vi "Draw Range Border.vi"(4 "Marker Options":T2={"Color"=16723218, "pen"={"Width"=2, "Style"=enum."Solid"}, "font"={"Font Name"="Arial", "Size"=16, "Strikeout?"=FALSE, "Italic?"=FALSE, "Underline?"=FALSE, "Outline?"=FALSE, "Shadow?"=FALSE, "Bold?"=FALSE, "FontColor"=0}, "caption"=""}, 6 "Type":T1, 7 "picture":picture, 9 "end Coords":T3, 10 "Plot Bounds":T4, 11 "Start Coords":T3) -> (5 "new picture":picture)   [LabVIEW 2014, in "Graph Extensions.lvlib"]
uses:
  Graph Extensions.lvlib
  <vilib>/Utility/miscctls.llb/LVRectTypeDef.ctl
  <vilib>/Utility/miscctls.llb/LVPoint32TypeDef.ctl
  controls/MarkerOptions.ctl
  controls/markerType.ctl
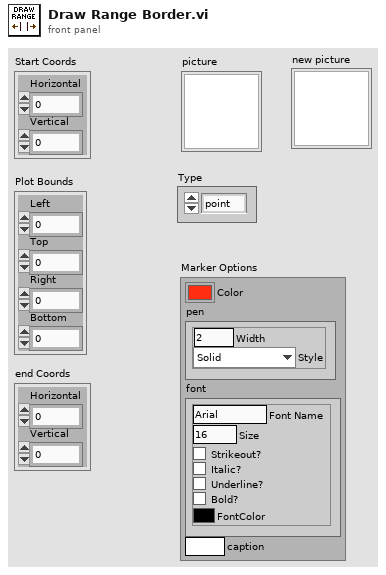
[diagram p1: front panel]
types:
  T1 = typedef "Graph Extensions.lvlib/markerType.ctl" = enum16{"point", "arrow", "horiz", "vert", "vert range", "horiz range", "box"}
  T2 = typedef "Graph Extensions.lvlib/MarkerOptions.ctl" = cluster{"Color":u32, "pen":cluster{"Width":u16, "Style":enum32{"Solid", "Dash", "Dot", "DashDot", "DashDotDot"}}, "font":cluster{"Font Name":string, "Size":i16, "Strikeout?":bool, "Italic?":bool, "Underline?":bool, "Outline?":bool, "Shadow?":bool, "Bold?":bool, "FontColor":u32}, "caption":string}
  T3 = typedef "LVPoint32TypeDef.ctl" = cluster{"Horizontal":i32, "Vertical":i32}
  T4 = typedef "LVRectTypeDef.ctl" = cluster{"Left":i16, "Top":i16, "Right":i16, "Bottom":i16}
  T5 = cluster{"Width":u16, "Style":enum32{"Solid", "Dash", "Dot", "DashDot", "DashDotDot"}}
  T6 = cluster{"left":i16, "top":i16, "right":i16, "bottom":i16}
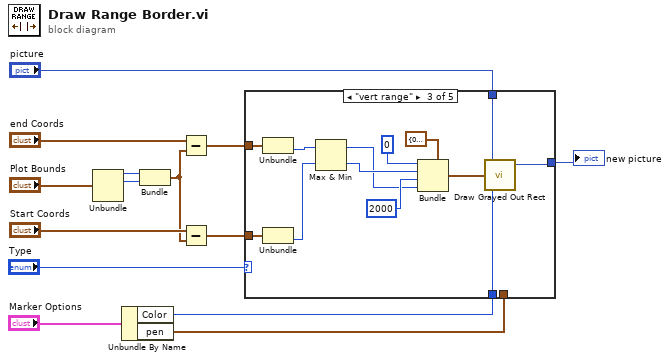
[diagram p0: block diagram]
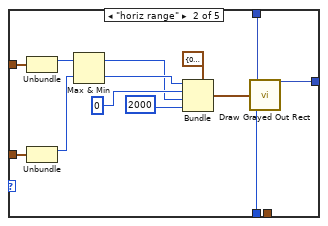
[diagram p3: hidden frame]
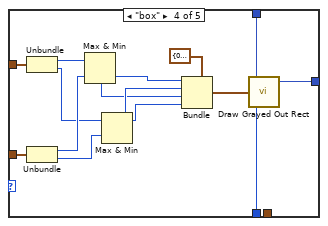
[diagram p4: hidden frame]
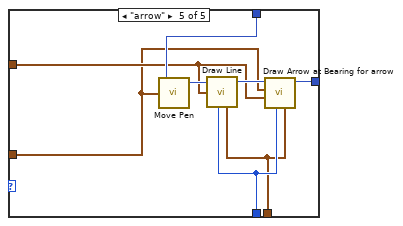
[diagram p5: hidden frame]
diagram:
  n1 = Unbundle("Plot Bounds") -> ("Left"=w14:i16, "Top"=w11:i16)  [unwired: 2 out]
  n2 = Unbundle By Name("Marker Options") -> ("Color"=w3:u32, "pen"=w1:T5)
  n3 = Bundle("Left"=w14, "Top"=w11) -> (w7:cluster{"Left":i16, "Top":i16})  [unwired: 1 in]
  n4 = Subtract(x="end Coords", y=w7) -> (x-y=w10:T3)
  n5 = Subtract(x="Start Coords", y=w7) -> (x-y=w9:T3)
  n6 = case shown="\"vert range\"" "Type" {
    tunnel: w10 -> [_ w26 w41 w54 w60]
    tunnel: w9 -> [_ w25 w40 w53 w58]
    tunnel: [w15 w22 w35 w45 w61] -> w4
    tunnel: w3 -> [_ w20 w33 w44 w59]
    tunnel: "picture" -> [w15 w21 w34 w43 w64]
    tunnel: w1 -> [_ _ _ _ w57]
    frame Default {
    }
    frame "horiz range" {
      n7 = Unbundle(w26) -> ("Horizontal"=w27:i32)  [unwired: 1 out]
      n8 = Unbundle(w25) -> ("Horizontal"=w28:i32)  [unwired: 1 out]
      n9 = Max & Min(x=w27, y=w28) -> (max(x,y)=w16:i32, min(x,y)=w17:i32)
      n10 = Bundle(cluster=T6 {"left"=0, "top"=0, "right"=0, "bottom"=0} ("rect"), "left"=w17, "top"=i16 0, "right"=w16, "bottom"=i16 2000 ("top")) -> (w24:T6)
      n11 = call <vilib>:"Draw Grayed Out Rect.vi"("color(black)"=w20, "rect"=w24, "picture"=w21) -> ("new picture"=w22:picture)  [unwired: 2 in]
    }
    frame "vert range" {
      n12 = Unbundle(w41) -> ("Vertical"=w39:i32)  [unwired: 1 out]
      n13 = Unbundle(w40) -> ("Vertical"=w38:i32)  [unwired: 1 out]
      n14 = Max & Min(x=w39, y=w38) -> (max(x,y)=w29:i32, min(x,y)=w30:i32)
      n15 = Bundle(cluster=T6 {"left"=0, "top"=0, "right"=0, "bottom"=0} ("rect"), "left"=i16 0 ("top"), "top"=w30, "right"=i16 2000 ("top"), "bottom"=w29) -> (w37:T6)
      n16 = call <vilib>:"Draw Grayed Out Rect.vi"("color(black)"=w33, "rect"=w37, "picture"=w34) -> ("new picture"=w35:picture)  [unwired: 2 in]
    }
    frame "box" {
      n17 = Unbundle(w54) -> ("Horizontal"=w55:i32, "Vertical"=w51:i32)
      n18 = Unbundle(w53) -> ("Horizontal"=w56:i32, "Vertical"=w52:i32)
      n19 = Max & Min(x=w55, y=w56) -> (max(x,y)=w48:i32, min(x,y)=w50:i32)
      n20 = Max & Min(x=w51, y=w52) -> (max(x,y)=w47:i32, min(x,y)=w49:i32)
      n21 = Bundle(cluster=T6 {"left"=0, "top"=0, "right"=0, "bottom"=0} ("rect"), "left"=w50, "top"=w49, "right"=w48, "bottom"=w47) -> (w46:T6)
      n22 = call <vilib>:"Draw Grayed Out Rect.vi"("color(black)"=w44, "rect"=w46, "picture"=w43) -> ("new picture"=w45:picture)  [unwired: 2 in]
    }
    frame "arrow" {
      n23 = call <vilib>:"Move Pen.vi"("new position"=w58, "picture"=w64) -> ("new picture"=w63:picture)  [unwired: 3 in]
      n24 = call <vilib>:"Draw Line.vi"("picture"=w63, "end point"=w60, "color(black)"=w59, "pen"=w57) -> ("new picture"=w62:picture)  [unwired: 5 in]
      n25 = call "Draw Arrow at Bearing for arrow.vi"("pen"=w57, "color(black)"=w59, "P2"=w60, "P1"=w58, "new picture in"=w62) -> ("new picture out"=w61:picture)  [unwired: 6 in]
    }
  }
  "new picture" <- w4
